vi "BAE6.vi"() -> ()   [LabVIEW 2014]
doc: "Front Panel View Manipulation BAE6\n\nChanges the position of this Vi's front panel from the center to the upper left corner of the screen through user input and updates and displays the window boundaries after each transition.\n\nBeverly Abadines\nPHY 350\nE6"
panel:
  out "Front Panel.WinBounds":T1
  out "position status":enum16{"center", "upper left"}(ring)
  in  "stop":bool
  in  "center":bool
  in  "upper left":bool
  # "FP View Manipulation"
  # "Beverly Abadines\nPhys 350\nE6"
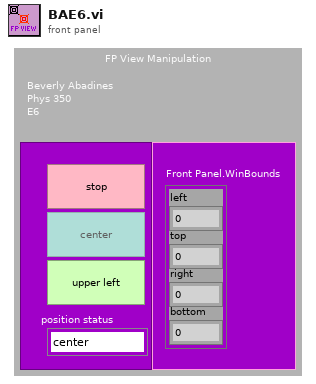
[diagram p1: front panel]
types:
  T1 = cluster{"left":i16, "top":i16, "right":i16, "bottom":i16}
  T2 = enum8{"Enabled", "Disabled", "Disabled and Grayed Out"}
  T3 = typedef "LVRectTypeDef.ctl" = cluster{"Left":i16, "Top":i16, "Right":i16, "Bottom":i16}
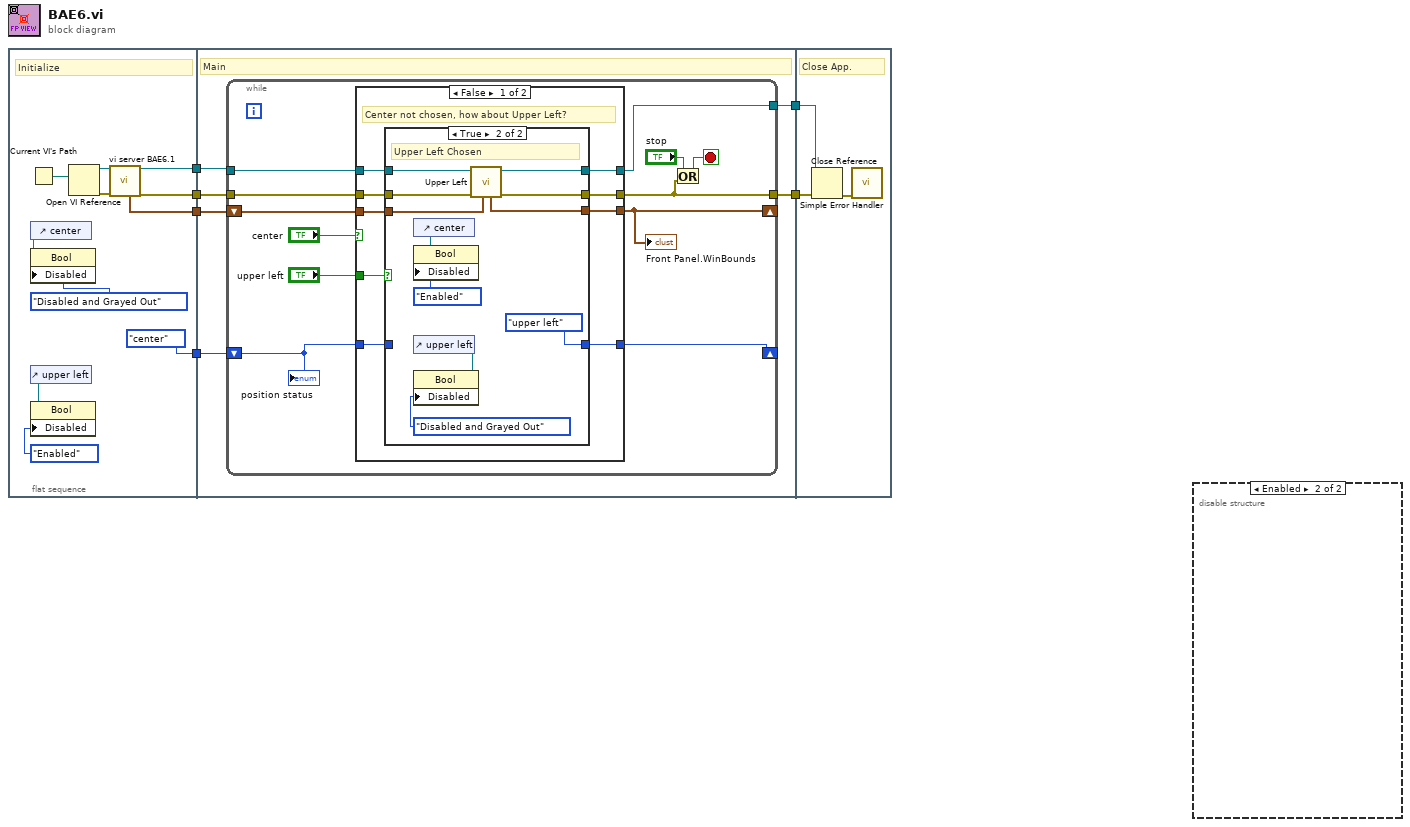
[diagram p0: block diagram]
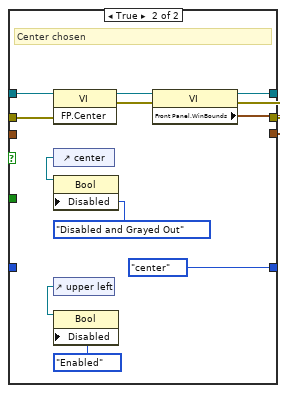
[diagram p3: hidden frame]
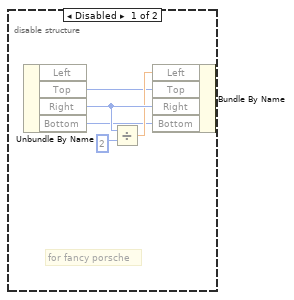
[diagram p4: hidden frame]
diagram:
  n1 = flat-sequence {
    tunnel: [w17] -> w6
    tunnel: [w16] -> w5
    tunnel: [w15] -> w4
    tunnel: [enum16{"center", "upper left"}."center" ("position status 2")] -> w3
    tunnel: w6 -> [w23]
    tunnel: w5 -> [w22]
    tunnel: w4 -> [w19]
    tunnel: w3 -> [w18]
    tunnel: [w21] -> w2
    tunnel: [w20] -> w1
    tunnel: w2 -> [w72]
    tunnel: w1 -> [w73]
    frame #0 {
      # "Initialize"
      n2 = Current VI's Path() -> (path=w14:path)
      n3 = control-ref of="center"() -> (w10:refnum<vi>)
      n4 = property class="Bool"(reference=w10, "Disabled"=T2."Disabled and Grayed Out") -> ()  [unwired: 1 in, 2 out]
      n5 = control-ref of="upper left"() -> (w8:refnum<vi>)
      n6 = property class="Bool"(reference=w8, "Disabled"=T2."Enabled") -> ()  [unwired: 1 in, 2 out]
      n7 = Open VI Reference(vi path=w14) -> (vi reference=w12:refnum<vi>, error out=w13:errorcluster)  [unwired: 5 in]
      n8 = call "vi server BAE6.1.vi"("VI ref in"=w12, "error in"=w13) -> ("VI ref out"=w17:refnum<vi>, "FP.WinBounds"=w15:T3, "error out"=w16:errorcluster)  [unwired: 11 in]
    }
    frame #1 {
      # "Main"
      n9 = while {
        tunnel: w23 -> [w34]
        tunnel: w22 -> [w33]
        tunnel: [w26] -> w21
        tunnel: [w31] -> w20
        shift-right: [w30] -> _
        shift-left: w18 -> [w24]
        shift-right: [w28] -> _
        shift-left: w19 -> [w32]
        stop <- w25 stop-if-true
        n10 = case shown="False" "center" {
          tunnel: w34 -> [w43 w65]
          tunnel: w33 -> [w42 w64]
          tunnel: w32 -> [w41 _]
          tunnel: [w38 w63] -> w31
          tunnel: [w39 w62] -> w26
          tunnel: [w40 w61] -> w28
          tunnel: [w37 enum16{"center", "upper left"}."center" ("position status 2")] -> w30
          tunnel: "upper left" -> [w44 _]
          tunnel: w24 -> [w36 _]
          frame False {
            # "Center not chosen, how about Upper Left?"
            n11 = case shown="True" w44 {
              tunnel: w43 -> [w48 w57]
              tunnel: w42 -> [w46 w56]
              tunnel: w41 -> [w47 w55]
              tunnel: [w47 w54] -> w40
              tunnel: [w46 w53] -> w39
              tunnel: [w48 w52] -> w38
              tunnel: [w45 enum16{"center", "upper left"}."upper left" ("position status 2")] -> w37
              tunnel: w36 -> [w45 _]
              frame False {
                # "Upper Left not chosen"
              }
              frame True {
                # "Upper Left Chosen"
                n12 = control-ref of="center"() -> (w49:refnum<vi>)
                n13 = property class="Bool"(reference=w49, "Disabled"=T2."Enabled") -> ()  [unwired: 1 in, 2 out]
                n14 = control-ref of="upper left"() -> (w58:refnum<vi>)
                n15 = property class="Bool"(reference=w58, "Disabled"=T2."Disabled and Grayed Out") -> ()  [unwired: 1 in, 2 out]
                n16 = call "Upper Left.vi"("VI in"=w57, "error in"=w56, "FP.WinBounds In"=w55) -> ("FP.WinBounds Out"=w54:T3, "ref out"=w52:refnum<vi>, "error out"=w53:errorcluster)  [unwired: 5 in]
              }
            }
          }
          frame True {
            # "Center chosen"
            n17 = invoke class="VI" method="FP.Center"(reference=w65, error in=w64) -> (reference out=w71:refnum<vi>, error out=w70:errorcluster)  [unwired: 1 in, 1 out]
            n18 = control-ref of="center"() -> (w66:refnum<vi>)
            n19 = property class="Bool"(reference=w66, "Disabled"=T2."Disabled and Grayed Out") -> ()  [unwired: 1 in, 2 out]
            n20 = control-ref of="upper left"() -> (w68:refnum<vi>)
            n21 = property class="Bool"(reference=w68, "Disabled"=T2."Enabled") -> ()  [unwired: 1 in, 2 out]
            n22 = property class="VI"(reference=w71, error in=w70) -> (reference out=w63:refnum<vi>, error out=w62:errorcluster, "Front Panel.WinBounds"=w61:T3)
          }
        }
        "Front Panel.WinBounds" <- w28
        n23 = Or(x="stop", y=w26) -> (x .or. y?=w25:bool)
        "position status" <- w24
      }
    }
    frame #2 {
      # "Close App."
      n24 = Close Reference ("Close LV Object Reference")(reference=w73, error in (no error)=w72) -> (error out=w74:errorcluster)
      n25 = call <vilib>:"Simple Error Handler.vi"("error in (no error)"=w74) -> ()  [unwired: 4 in, 5 out]
    }
  }
  n26 = disable-structure shown="Enabled" {
    frame Disabled {
      # "for fancy porsche"
      n27 = Unbundle By Name() -> ("Top"=w77:i16, "Right"=w80:i16, "Bottom"=w75:i16)  [unwired: 1 in, 1 out]
      n28 = Divide(x=w80, y=i16 2) -> (x/y=w79:dbl)
      n29 = Bundle By Name("Left"=w79, "Top"=w77, "Right"=w80, "Bottom"=w75) -> (w81:cluster{}, w78:cluster{})
    }
    frame Enabled {
    }
  }
